vi "Main Menu.vi"() -> ()   [LabVIEW 2020]
panel:
  out "error out":errorcluster
  in  "Step Size (seconds)":dbl=0.01 min=0.01 max=1.0 step=0.05
  in  "Window Size (seconds)":dbl=0.01 min=0.01 max=1.0 step=0.05
  in  "Run Button":bool
  in  "Open Button":bool
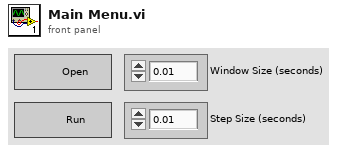
[diagram p1: front panel]
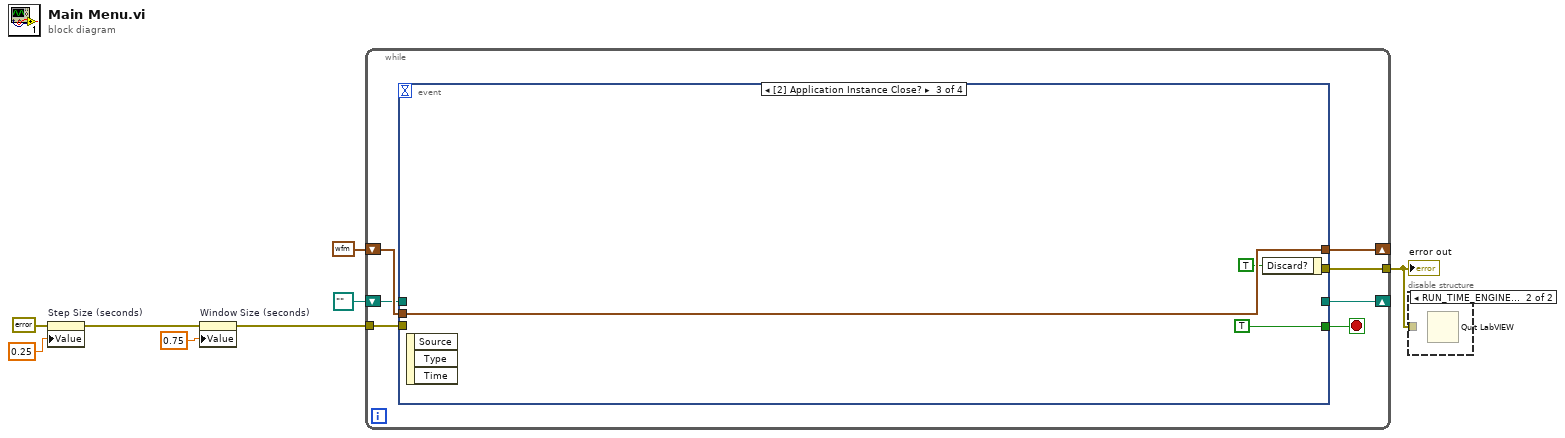
[diagram p0: block diagram]
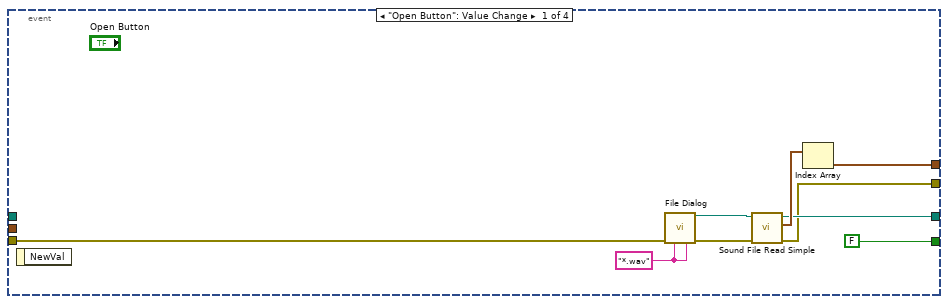
[diagram p3: hidden frame]
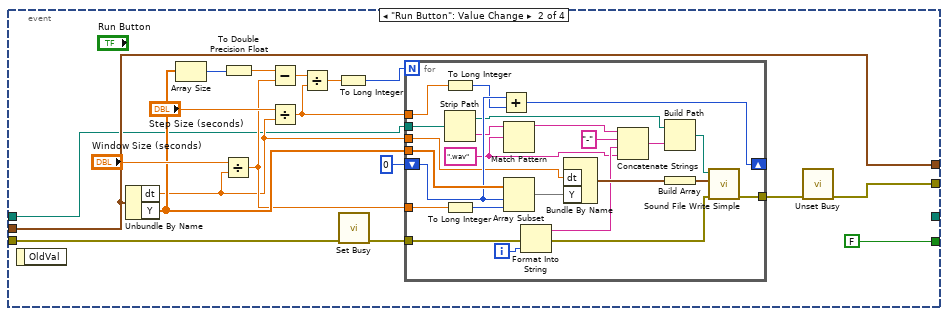
[diagram p4: hidden frame]
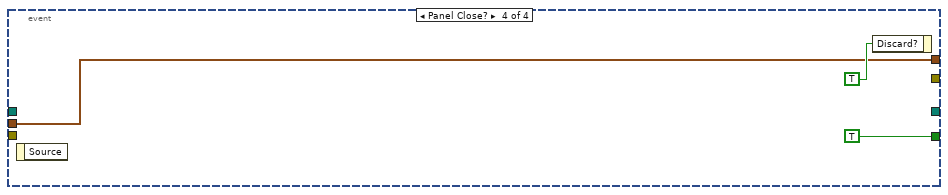
[diagram p5: hidden frame]
diagram:
  n1 = property on="Step Size (seconds)" class="DigNum (strict)"(error in=errorcluster {"status"=FALSE, "code"=0, "source"=""} ("error in (no error)"), "Value"=0.25 ("Step Size (seconds)")) -> (error out=w4:errorcluster)  [unwired: 1 in, 1 out]
  n2 = property on="Window Size (seconds)" class="DigNum (strict)"(error in=w4, "Value"=0.75 ("Window Size (seconds)")) -> (error out=w3:errorcluster)  [unwired: 1 in, 1 out]
  n3 = while {
    shift-right: [w14] -> _
    shift-left: waveform(dbl) {"t0"=timestamp(0 s since 1904-01-01), "dt"=1.0, "Y"=[]} ("element") -> [w13]
    shift-right: [w12] -> _
    shift-left: path "" ("path out") -> [w11]
    tunnel: w3 -> [w10]
    tunnel: [w9] -> w1
    stop <- w15 stop-if-true
    n4 = event shown="[2] Application Instance Close?" {
      selector: _ -> [_ _ _ _]
      dyn-events: _ -> [_ _ _ _]
      timeout: _ -> [_ _ _ _]
      tunnel: [FALSE FALSE TRUE TRUE] -> w15
      tunnel: [w19 w30 w69 w71] -> w14
      tunnel: w13 -> [_ w30 w69 w71]
      tunnel: [w18 _ _ _] -> w12
      tunnel: w11 -> [_ w29 _ _]
      tunnel: w10 -> [w17 w28 _ _]
      tunnel: [w16 w25 _ _] -> w9
      event "Open Button": Value Change {
        w23 = "*.wav" ("pattern label")
        n5 = event-data() -> ()  [unwired: 1 in, 1 out]
        n6 = call "File Dialog"("error in"=w17, "pattern (all files)"=w23, "pattern label"=w23) -> ("selected path"=w21:path, "error out"=w22:errorcluster)  [unwired: 9 in, 2 out]
        n7 = call <vilib>:"Sound File Read Simple.vi"("error in (no error)"=w22, "path"=w21) -> ("error out"=w16:errorcluster, "data"=w20:waveform(dbl)[], "path out"=w18:path)  [unwired: 6 in, 1 out]
        n8 = Index Array(array=w20) -> (element=w19:waveform(dbl))  [unwired: 1 in]
      }
      event "Run Button": Value Change {
        n9 = event-data() -> ()  [unwired: 1 in, 1 out]
        n10 = Unbundle By Name(w30) -> ("dt"=w31:dbl, "Y"=w35:dbl[])
        n11 = Array Size(array=w35) -> (size(s)=w40:i32)
        n12 = Divide(x="Window Size (seconds)", y=w31) -> (x/y=w34:dbl)
        n13 = To Double Precision Float(number=w40) -> (double precision float=w39:dbl)
        n14 = Subtract(x=w39, y=w34) -> (x-y=w38:dbl)
        n15 = Divide(x="Step Size (seconds)", y=w31) -> (x/y=w32:dbl)
        n16 = Divide(x=w38, y=w32) -> (x/y=w36:dbl)
        n17 = To Long Integer(number=w36) -> (32bit integer=w37:i32)
        n18 = call <vilib>:"Set Busy.vi"("error in (no error)"=w28) -> ("error out"=w27:errorcluster)  [unwired: 9 in, 1 out]
        n19 = for {
          N: w37 -> [_]
          tunnel: w35 -> [w67]
          tunnel: w34 -> [w65]
          shift-right: [w62] -> _
          shift-left: 0 -> [w64]
          tunnel: w32 -> [w61]
          tunnel: w31 -> [w59]
          tunnel: w29 -> [w56]
          tunnel: w27 -> [w47]
          tunnel: [w45] -> w26
          i -> [w44]
          w50 = ".wav" ("regular expression")
          n20 = To Long Integer(number=w61) -> (32bit integer=w63:i32)
          n21 = Strip Path(path=w56) -> (stripped path=w55:path, name=w54:string)
          n22 = To Long Integer(number=w65) -> (32bit integer=w66:i32)
          n23 = Add(x=w64, y=w63) -> (x+y=w62:i32)
          n24 = Match Pattern(string=w54, regular expression=w50) -> (before substring=w53:string)  [unwired: 1 in, 3 out]
          n25 = Array Subset(array=w67, index=w64, length=w66) -> (w60:dbl[])
          n26 = Format Into String(error in=w47, w44) -> (resulting string=w51:string, error out=w46:errorcluster)  [unwired: 2 in]
          n27 = Bundle By Name("dt"=w59, "Y"=w60) -> (w57:waveform(dbl))  [unwired: 1 in]
          n28 = Concatenate Strings(w53, "-" ("string"), w51, w50) -> (w49:string)
          n29 = Build Path(base path=w55, name or relative path=w49) -> (appended path=w48:path)
          n30 = Build Array(w57) -> (w58:waveform(dbl)[])
          n31 = call <vilib>:"Sound File Write Simple.vi"("error in (no error)"=w46, "data"=w58, "path"=w48) -> ("error out"=w45:errorcluster)  [unwired: 7 in, 1 out]
        }
        n32 = call <vilib>:"Unset Busy.vi"("error in (no error)"=w26) -> ("error out"=w25:errorcluster)  [unwired: 10 in]
      }
      event Application Instance Close? {
        n33 = event-data() -> ()  [unwired: 1 in, 3 out]
        n34 = event-data("Discard?"=TRUE) -> ()  [unwired: 1 in, 1 out]
      }
      event Panel Close? {
        n35 = event-data() -> ()  [unwired: 1 in, 1 out]
        n36 = event-data("Discard?"=TRUE) -> ()  [unwired: 1 in, 1 out]
      }
    }
  }
  "error out" <- w1
  n37 = disable-structure shown="RUN_TIME_ENGINE==True" {
    disable-tunnel: w1 -> [_ _]
    frame condition #0 (active) {
    }
    frame condition #1 {
      n38 = Quit LabVIEW() -> ()  [unwired: 1 in]
    }
  }
